vi "updateTrialInfo (SubVI).vi"(2 "data Path":path, 3 "pre Protocol":T1) -> (0 "file path out":path, 1 "next":T1)   [LabVIEW 2011]
uses:
  ctlProtocol.ctl
  ctlProtocolSubID.ctl
  ctlProtocolUnit.ctl
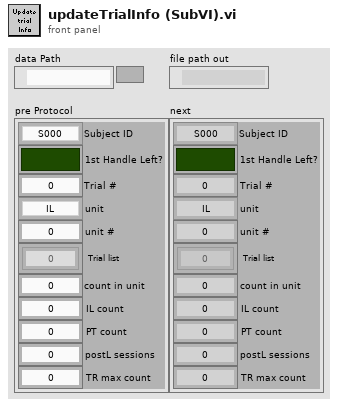
[diagram p1: front panel]
types:
  T1 = typedef "ctlProtocol.ctl" = cluster{"Subject ID":T2, "1st Handle Left?":bool, "Trial #":i32, "unit":T3, "unit #":i32, "Trial list":i32[], "count in unit":i32, "IL count":i32, "PT count":i32, "postL sessions":i32, "TR max count":i32}
  T2 = typedef "ctlProtocolSubID.ctl" = enum16{"S000", "S001", "S002", "S003", "S004", "S005", "S006", "S007", "S008", "S009", "S010", "S011", "S012", "S013", "S014", "S015", "S016", "S017", "S018", "S019", "S020", "S021", "S022", "S023", "S024", "S025", "S026", "S027", "S028", "S029", "S030", "S031", "S032", "S033", "S034", "S035", "S036", "S037", "S038", "S039", "S040"}
  T3 = typedef "ctlProtocolUnit.ctl" = enum16{"IL", "TR", "PT"}
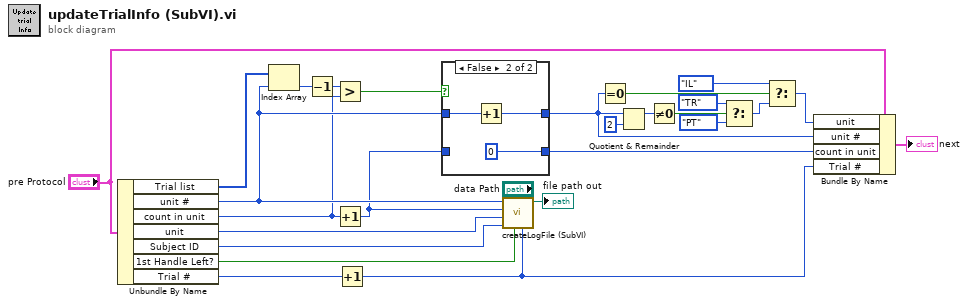
[diagram p0: block diagram]
diagram:
  n1 = Unbundle By Name("pre Protocol") -> ("Trial list"=w13:i32[], "unit #"=w11:i32, "count in unit"=w10:i32, "unit"=w5:T3, "Subject ID"=w6:T2, "1st Handle Left?"=w7:bool, "Trial #"=w4:i32)
  n2 = Index Array(array=w13, index=w11) -> (element=w26:i32)
  n3 = Decrement(x=w26) -> (x-1=w27:i32)
  n4 = Greater?(x=w27, y=w10) -> (0:w12:bool)
  n5 = Increment(x=w10) -> (x+1=w9:i32)
  n6 = Increment(x=w4) -> (x+1=w3:i32)
  n7 = case shown="False" w12 {
    tunnel: [w29 0 ("t")] -> w2
    tunnel: w9 -> [w29 _]
    tunnel: w11 -> [w28 w31]
    tunnel: [w28 w30] -> w14
    frame True {
    }
    frame False {
      n8 = Increment(x=w31) -> (x+1=w30:i32)
    }
  }
  n9 = call "createLogFile (SubVI).vi"("trial #"=w3, "1st Handle Left?"=w7, "directory Path"="data Path", "Subject ID"=w6, "unit"=w5, "count in unit"=w9, "unit #"=w11) -> ("file path out"=→"file path out":path)  [unwired: 3 in]
  n10 = Equal To 0?(x=w14) -> (x = 0?=w23:bool)
  n11 = Quotient & Remainder(x=w14, y=2) -> (x-y*floor(x/y)=w19:i32)  [unwired: 1 out]
  n12 = Not Equal To 0?(x=w19) -> (x != 0?=w20:bool)
  n13 = Select(t=ctlProtocolUnit."TR" ("Protocol.unit"), s=w20, f=ctlProtocolUnit."PT" ("Protocol.unit")) -> (s? t:f=w25:T3)
  n14 = Select(t=ctlProtocolUnit."IL" ("Protocol.unit"), s=w23, f=w25) -> (s? t:f=w15:T3)
  n15 = Bundle By Name(cluster="pre Protocol", "unit"=w15, "unit #"=w14, "count in unit"=w2, "Trial #"=w3) -> (→"next":T1)
